vi "Get Corner Mask.vi"(8 "Error In":errorcluster, 10 "Blue Channel In":T1(plugin-control), 11 "Red Channel In":T1(plugin-control)) -> (0 "Error Out":errorcluster, 1 "Corner Mask":T1(plugin-control), 2 "Blue Channel Out":T1(plugin-control), 3 "Red Channel Out":T1(plugin-control))   [LabVIEW 2018]
uses:
  <vilib>/vision/NI_Vision_Development_Module.lvlib
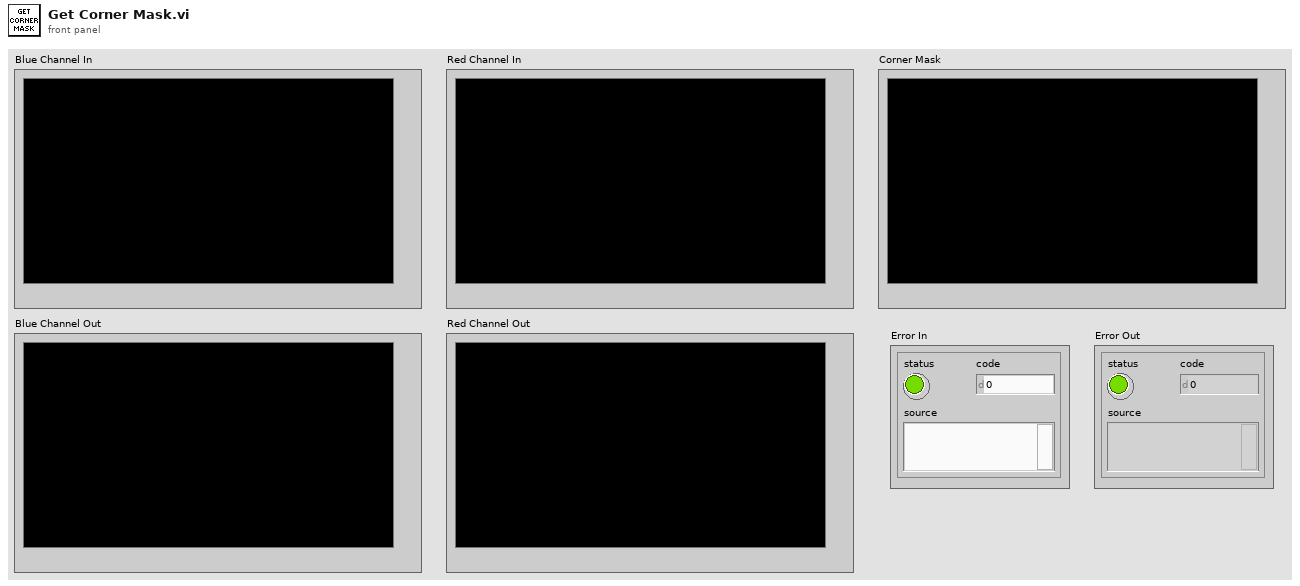
[diagram p1: front panel]
types:
  T1 = typedef "IMAQ Image.ctl" = refnum<image>
  T2 = cluster{"Global Rectangle":i32[], "Contours":cluster{"Contour Type":u32, "ROI Type":u32, "Points":i32[]}[]}
  T3 = cluster{"Contour Type":u32, "ROI Type":u32, "Points":i32[]}[]
  T4 = cluster{"Contour Type":u32, "ROI Type":u32, "Points":i32[]}
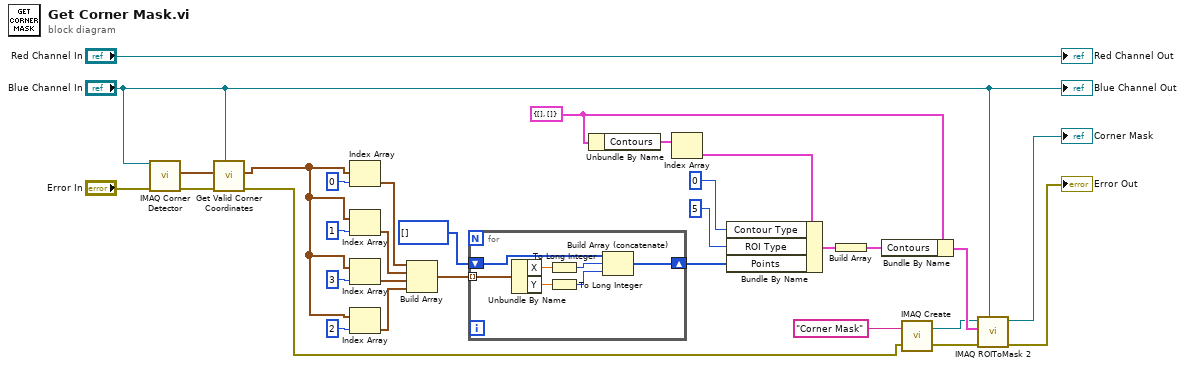
[diagram p0: block diagram]
diagram:
  w19 = T2 {"Global Rectangle"=[], "Contours"=[]} ("ROI")
  n1 = call "IMAQ Corner Detector"("Image"="Blue Channel In", "error in (no error)"="Error In") -> ("Corner Point Coordinates"=w28:cluster{"X":sgl, "Y":sgl}[], "error out"=w29:errorcluster)  [unwired: 8 in, 4 out]
  n2 = call "Get Valid Corner Coordinates.vi"("Reference Image"="Blue Channel In", "Error In"=w29, "Coordinates"=w28) -> ("Error Out"=w6:errorcluster, "Corners"=w3:cluster{"X":sgl, "Y":sgl}[])  [unwired: 7 in]
  n3 = Index Array(array=w3, index=0) -> (element=w24:cluster{"X":sgl, "Y":sgl})
  n4 = Index Array(array=w3, index=1) -> (element=w25:cluster{"X":sgl, "Y":sgl})
  n5 = Index Array(array=w3, index=3) -> (element=w26:cluster{"X":sgl, "Y":sgl})
  n6 = Index Array(array=w3, index=2) -> (element=w27:cluster{"X":sgl, "Y":sgl})
  n7 = Build Array(w24, w25, w26, w27) -> (w2:cluster{"X":sgl, "Y":sgl}[])
  n8 = for {
    shift-right: [w35] -> w15
    shift-left: i32[] [] -> [w38]
    tunnel: w2 -> [w34] mode=indexing
    n9 = Unbundle By Name(w34) -> ("X"=w32:sgl, "Y"=w33:sgl)
    n10 = To Long Integer(number=w32) -> (32bit integer=w37:i32)
    n11 = To Long Integer(number=w33) -> (32bit integer=w36:i32)
    n12 = Build Array (concatenate)(w38, w37, w36) -> (w35:i32[])
  }
  n13 = Unbundle By Name(w19) -> ("Contours"=w11:T3)
  n14 = Index Array(array=w11) -> (element=w12:T4)  [unwired: 1 in]
  n15 = Bundle By Name(cluster=w12, "Contour Type"=u32 0, "ROI Type"=u32 5, "Points"=w15) -> (w16:T4)
  n16 = Build Array(w16) -> (w17:T3)
  n17 = Bundle By Name(cluster=w19, "Contours"=w17) -> (w18:T2)
  n18 = call "IMAQ Create"("Image Name"="Corner Mask", "error in (no error)"=w6) -> ("New Image"=w9:T1, "error out"=w7:errorcluster)  [unwired: 3 in]
  n19 = call "IMAQ ROIToMask 2"("Image Model"="Blue Channel In", "error in (no error)"=w7, "ROI Descriptor"=w18, "Image"=w9) -> ("error out"=→"Error Out":errorcluster, "Image Out"=→"Corner Mask":T1)  [unwired: 5 in, 1 out]
  "Blue Channel Out" <- "Blue Channel In"
  "Red Channel Out" <- "Red Channel In"
